vi "ExSubCreateFileNDataHandles.vi"(2 "error in (no error)":errorcluster, 3 "File and Display Name":string, 4 "Camera Handle":u32) -> (0 "error out":errorcluster, 1 "Handles Out":T1)   [LabVIEW 2010]
panel:
  # "ExSubCreateFileNDataHandles:\nThis is a SubVI that creates file and image \nobjects and returns the handles bundled in a cluster \nthat includes a camera handle"
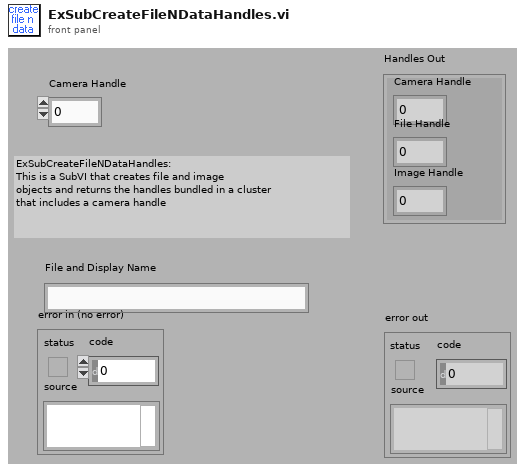
[diagram p1: front panel]
types:
  T1 = cluster{"Camera Handle":u32, "File Handle":u32, "Image Handle":u32}
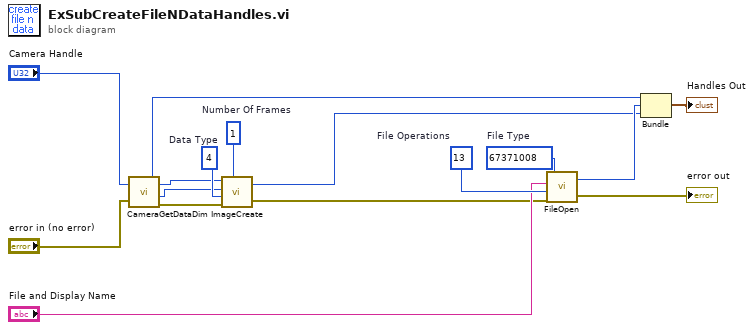
[diagram p0: block diagram]
diagram:
  w6 = u32 1  # Number Of Frames
  w7 = u32 4  # Data Type
  w9 = 13  # File Operations
  w10 = 67371008  # File Type
  n1 = call <userlib>:"CameraGetDataDim.vi"("Camera Handle"="Camera Handle", "error in"="error in (no error)") -> ("Camera Handle"=w12:u32, "Xdim"=w3:u32, "Ydim"=w2:u32, "error out"=w16:errorcluster)
  n2 = call <userlib>:"ImageCreate.vi"("X dimension"=w3, "Y dimension"=w2, "Data Type"=w7, "error in"=w16, "Number Of Frames"=w6) -> ("Image Handle"=w1:u32, "error out"=w4:errorcluster)
  n3 = call <userlib>:"FileOpen.vi"("error in"=w4, "File Operations"=w9, "FileName"="File and Display Name", "File Type"=w10) -> ("error out"=→"error out":errorcluster, "File Handle"=w11:u32)
  n4 = Bundle("Camera Handle"=w12, "File Handle"=w11, "Image Handle"=w1) -> (→"Handles Out":T1)  [unwired: 1 in]
